vi "Set Indicators Visibility Status.vi"(10 "Indicator Refs":refnum<vi>[](array[refnum]), 11 "Label":string) -> ()   [LabVIEW 2021, in "Panther Dashboard.lvlib"]
uses:
  Panther Dashboard.lvlib
  <vilib>/Utility/miscctls.llb/LVPositionTypeDef.ctl
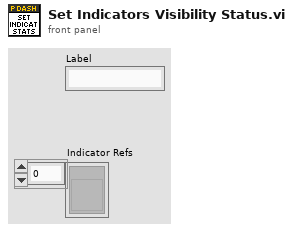
[diagram p1: front panel]
types:
  T1 = typedef "LVPositionTypeDef.ctl" = cluster{"Left":i32, "Top":i32}
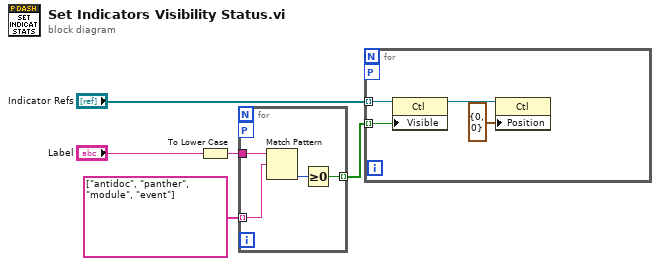
[diagram p0: block diagram]
diagram:
  n1 = To Lower Case(string="Label") -> (all lower case string=w1:string)
  n2 = for {
    tunnel: [w9] -> w5 mode=indexing
    tunnel: string[] ["antidoc", "panther", "module", "event"] ("regular expression") -> [w7] mode=indexing
    tunnel: w1 -> [w6]
    workers-P: _ -> [_]
    n3 = Match Pattern(string=w6, regular expression=w7) -> (offset past match=w8:i32)  [unwired: 1 in, 3 out]
    n4 = Greater Or Equal To 0?(x=w8) -> (x >= 0?=w9:bool)
  }
  n5 = for {
    tunnel: w5 -> [w13] mode=indexing
    tunnel: "Indicator Refs" -> [w12] mode=indexing
    workers-P: _ -> [_]
    n6 = property on="Property Node" class="Ctl"(reference=w12, "Visible"=w13) -> (reference out=w11:refnum<vi>)  [unwired: 1 in, 1 out]
    n7 = property on="Property Node" class="Ctl"(reference=w11, "Position"=T1 {"Left"=0, "Top"=0}) -> ()  [unwired: 1 in, 2 out]
  }
